vi "GUI-Get Set A FP Ctrl & Indi Value.vi"(0 "All Object Ref":refnum<vi>[](array[refnum]), 2 "Label":string, 5 "All Object Label":string[](array[string]), 7 "Ctrl Value In":variant, 13 "Set(F)":bool) -> (4 "Ctl Refnum":refnum<vi>, 6 "Refnum OK?":bool, 8 "Ctrl Value Out":variant, 15 "error out":errorcluster)   [LabVIEW 2024]
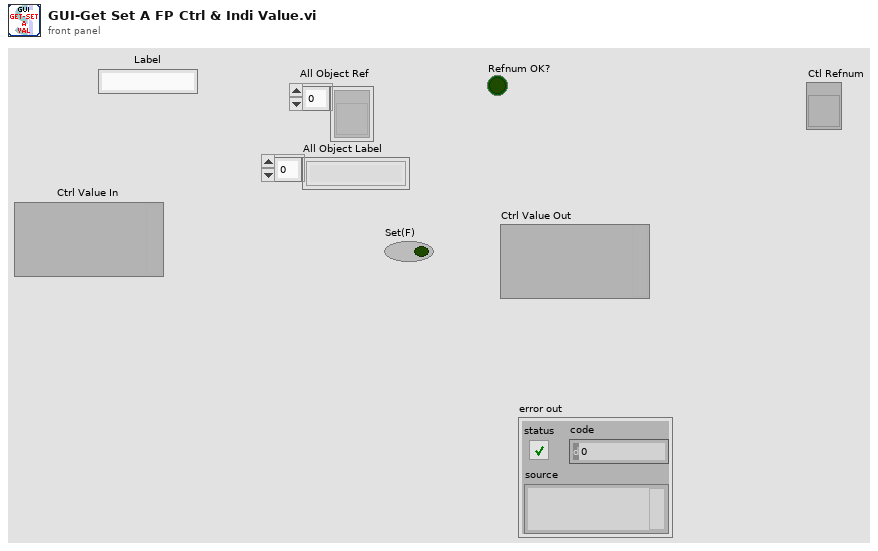
[diagram p1: front panel]
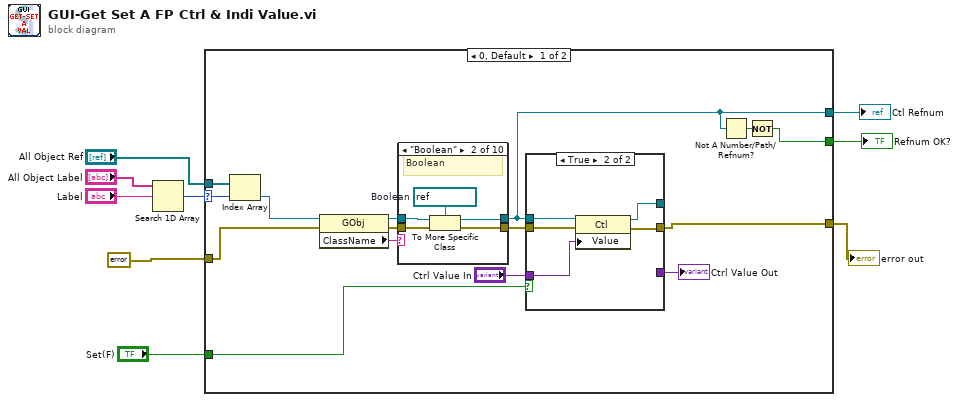
[diagram p0: block diagram]
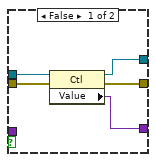
[diagram p2: hidden frame]
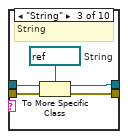
[diagram p4: hidden frame]
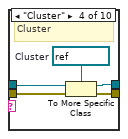
[diagram p5: hidden frame]
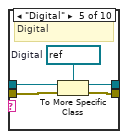
[diagram p6: hidden frame]
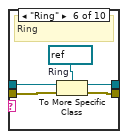
[diagram p7: hidden frame]
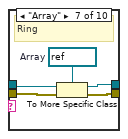
[diagram p8: hidden frame]
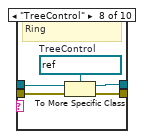
[diagram p9: hidden frame]
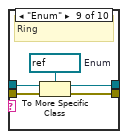
[diagram p10: hidden frame]
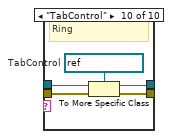
[diagram p11: hidden frame]
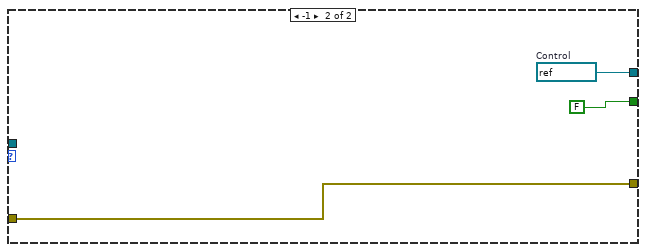
[diagram p12: hidden frame]
diagram:
  n1 = Search 1D Array(1D array="All Object Label", element="Label") -> (index of element=w4:i32)  [unwired: 1 in]
  n2 = case shown="0, Default" w4 {
    selector: w4 -> [w16 _]
    tunnel: "Set(F)" -> [w24 _]
    tunnel: errorcluster {"status"=FALSE, "code"=0, "source"=""} ("error in (no error)") -> [w12 w83]
    tunnel: [w10 w83] -> w8
    tunnel: "All Object Ref" -> [w17 _]
    tunnel: [w14 w82] -> w3
    tunnel: [w11 FALSE] -> w2
    frame 0, Default {
      n3 = Index Array(array=w17, index=w16) -> (element=w15:refnum<vi>)
      n4 = property class="GObj"(reference=w15, error in=w12) -> (reference out=w22:refnum<vi>, error out=w21:errorcluster, "ClassName"=w23:string)
      n5 = case shown="\"Boolean\"" w23 {
        tunnel: w22 -> [_ w40 w45 w50 w55 w60 w65 w70 w75 w80]
        tunnel: [_ w36 w43 w48 w52 w58 w63 w68 w73 w77] -> w14
        tunnel: w21 -> [w35 w38 w42 w47 w53 w57 w62 w67 w72 w78]
        tunnel: [w35 w37 w41 w46 w51 w56 w61 w66 w71 w76] -> w20
        frame Default {
        }
        frame "Boolean" {
          w39 = refnum<vi> refnum  # Boolean
          # "Boolean"
          n6 = To More Specific Class(target class=w39, reference=w40, error in=w38) -> (specific class reference=w36:refnum<vi>, error out=w37:errorcluster)
        }
        frame "String" {
          w44 = refnum<vi> refnum  # String
          # "String"
          n7 = To More Specific Class(target class=w44, reference=w45, error in=w42) -> (specific class reference=w43:refnum<vi>, error out=w41:errorcluster)
        }
        frame "Cluster" {
          w49 = refnum<vi> refnum  # Cluster
          # "Cluster"
          n8 = To More Specific Class(target class=w49, reference=w50, error in=w47) -> (specific class reference=w48:refnum<vi>, error out=w46:errorcluster)
        }
        frame "Digital" {
          w54 = refnum<vi> refnum  # Digital
          # "Digital"
          n9 = To More Specific Class(target class=w54, reference=w55, error in=w53) -> (specific class reference=w52:refnum<vi>, error out=w51:errorcluster)
        }
        frame "Ring" {
          w59 = refnum<vi> refnum  # Ring
          # "Ring"
          n10 = To More Specific Class(target class=w59, reference=w60, error in=w57) -> (specific class reference=w58:refnum<vi>, error out=w56:errorcluster)
        }
        frame "Array" {
          w64 = refnum<vi> refnum  # Array
          # "Ring"
          n11 = To More Specific Class(target class=w64, reference=w65, error in=w62) -> (specific class reference=w63:refnum<vi>, error out=w61:errorcluster)
        }
        frame "TreeControl" {
          w69 = refnum<vi> refnum  # TreeControl
          # "Ring"
          n12 = To More Specific Class(target class=w69, reference=w70, error in=w67) -> (specific class reference=w68:refnum<vi>, error out=w66:errorcluster)
        }
        frame "Enum" {
          w74 = refnum<vi> refnum  # Enum
          # "Ring"
          n13 = To More Specific Class(target class=w74, reference=w75, error in=w72) -> (specific class reference=w73:refnum<vi>, error out=w71:errorcluster)
        }
        frame "TabControl" {
          w79 = refnum<vi> refnum  # TabControl
          # "Ring"
          n14 = To More Specific Class(target class=w79, reference=w80, error in=w78) -> (specific class reference=w77:refnum<vi>, error out=w76:errorcluster)
        }
      }
      n15 = case shown="True" w24 {
        tunnel: w14 -> [w29 w34]
        tunnel: w20 -> [w28 w31]
        tunnel: [w27 w32] -> _
        tunnel: [w26 w33] -> w10
        tunnel: [w25 _] -> w19
        tunnel: "Ctrl Value In" -> [_ w30]
        frame False {
          n16 = property class="Ctl"(reference=w29, error in=w28) -> (reference out=w27:refnum<vi>, error out=w26:errorcluster, "Value"=w25:variant)
        }
        frame True {
          n17 = property class="Ctl"(reference=w34, error in=w31, "Value"=w30) -> (reference out=w32:refnum<vi>, error out=w33:errorcluster)
        }
      }
      "Ctrl Value Out" <- w19
      n18 = Not A Number/Path/Refnum?(number/path/refnum=w14) -> (NaN/Path/Refnum?=w13:bool)
      n19 = Not(x=w13) -> (.not. x?=w11:bool)
    }
    frame -1 {
      w82 = refnum<vi> refnum  # Control
    }
  }
  "error out" <- w8
  "Ctl Refnum" <- w3
  "Refnum OK?" <- w2
